vi "Choreo_TrajectoryCacheDifferential_New.vi"(8 "error in (no error)":errorcluster) -> (0 "error out":errorcluster)   [LabVIEW 2019, in "ChoreoLib.lvlib"]
doc: "Initialize and clear the differential trajectory memory cache\n\nInputs:\n -- ErrorIn -- cluster -- standard error cluster. Can be used to force execution sequence.\n\nOutputs:\n -- ErrorOut -- cluster -- standard error cluster. Can be used to force execution sequence and check for error."
uses:
  ChoreoLib.lvlib
  TypeDef/ChoreoTrajectoryCacheDifferential.ctl
  TypeDef/ChoreoTrajectoryDifferential.ctl
  TypeDef/ChoreoDifferentialSample.ctl
  TypeDef/ChoreoEventMarker.ctl
  Choreo_Choreo_Globals.vi
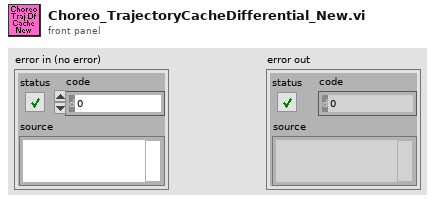
[diagram p1: front panel]
types:
  T1 = typedef "ChoreoLib.lvlib/ChoreoTrajectoryCacheDifferential.ctl" = map{string, T2}
  T2 = typedef "ChoreoLib.lvlib/ChoreoTrajectoryDifferential.ctl" = cluster{"name":string, "samples":T3[], "splits":i32[], "events":T4[]}
  T3 = typedef "ChoreoLib.lvlib/ChoreoDifferentialSample.ctl" = cluster{"timestamp":dbl, "x":dbl, "y":dbl, "heading":dbl, "velocityL":dbl, "velocityR":dbl, "angularVelocity":dbl, "accelL":dbl, "accelR":dbl, "accelAngular":dbl, "forceL":dbl, "forceR":dbl}
  T4 = typedef "ChoreoLib.lvlib/ChoreoEventMarker.ctl" = cluster{"TimeStamp":dbl, "Name":string}
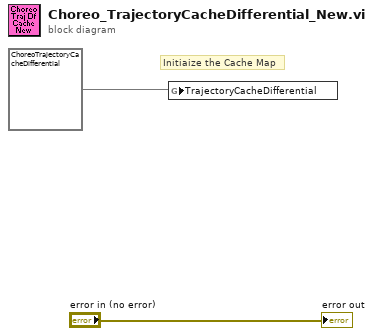
[diagram p0: block diagram]
diagram:
  # "Initiaize the Cache Map"
  n1 = global write "Choreo_Choreo_Globals.vi" "TrajectoryCacheDifferential"(T1 {} ("TrajectoryCacheDifferential")) -> ()
  "error out" <- "error in (no error)"
